vi "Add_OP.vi"() -> (2 "ADD/OP":T1, 3 "Cancel 2":bool)   [LabVIEW 2024]
panel:
  in  "Cancel":bool
  in  "Add":bool
  in  "PASSWORD:":string
  in  "OPERATOR NAME:":string
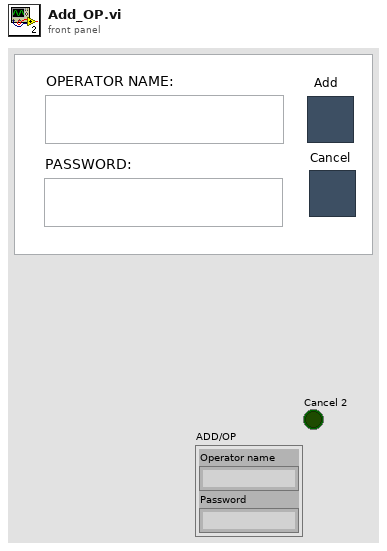
[diagram p1: front panel]
types:
  T1 = cluster{"Operator name":string, "Password":string}
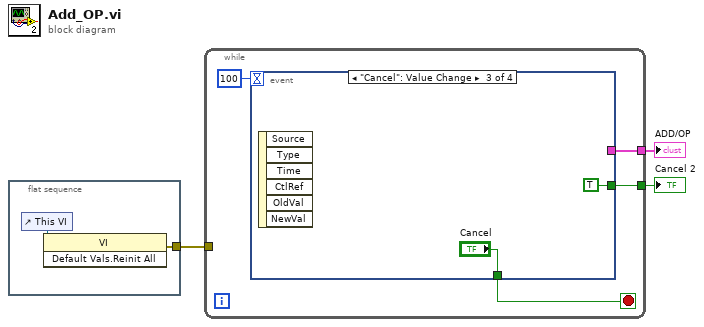
[diagram p0: block diagram]
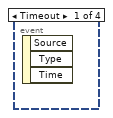
[diagram p2: hidden frame]
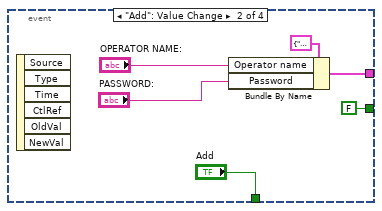
[diagram p3: hidden frame]
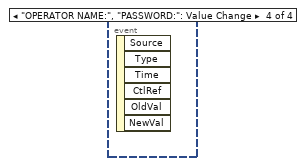
[diagram p4: hidden frame]
diagram:
  n1 = flat-sequence {
    tunnel: [w4] -> w1
    frame #0 {
      n2 = control-ref of="This VI"() -> (w5:refnum<vi>)
      n3 = invoke class="VI" method="Default Vals.Reinit All"(reference=w5) -> (error out=w4:errorcluster)  [unwired: 2 in, 2 out]
    }
  }
  n4 = while {
    tunnel: [w7] -> w3
    tunnel: [w6] -> w2
    tunnel: w1 -> [_]
    stop <- w8 stop-if-true
    n5 = event shown="[2] \"Cancel\": Value Change" {
      selector: _ -> [_ _ _ _]
      dyn-events: _ -> [_ _ _ _]
      timeout: 100 -> [_ _ _ _]
      tunnel: [_ "Add" "Cancel" _] -> w8
      tunnel: [_ w11 _ _] -> w7
      tunnel: [_ FALSE ("Cancel") TRUE ("Cancel") _] -> w6
      event Timeout {
        n6 = event-data() -> ()  [unwired: 1 in, 3 out]
      }
      event "Add": Value Change {
        n7 = event-data() -> ()  [unwired: 1 in, 6 out]
        n8 = Bundle By Name(cluster=T1 {"Operator name"="", "Password"=""} ("Cluster"), "Operator name"="OPERATOR NAME:", "Password"="PASSWORD:") -> (w11:T1)
      }
      event "Cancel": Value Change {
        n9 = event-data() -> ()  [unwired: 1 in, 6 out]
      }
      event "OPERATOR NAME:", "PASSWORD:": Value Change {
        n10 = event-data() -> ()  [unwired: 1 in, 6 out]
      }
    }
  }
  "ADD/OP" <- w3
  "Cancel 2" <- w2
